vi "Add Element in Array Guidance.vi"(8 "error in (no error)":errorcluster, 10 "Guidance input":refnum<class "Guidance.lvclass">, 11 "Vessel in":refnum<class "Vessel.lvclass">) -> (0 "error out":errorcluster, 2 "Index":i32, 3 "Vessel out":refnum<class "Vessel.lvclass">)   [LabVIEW 2014, in "Vessel.lvclass"]
uses:
  Vessel.lvclass
  Guidance/Guidance.lvclass
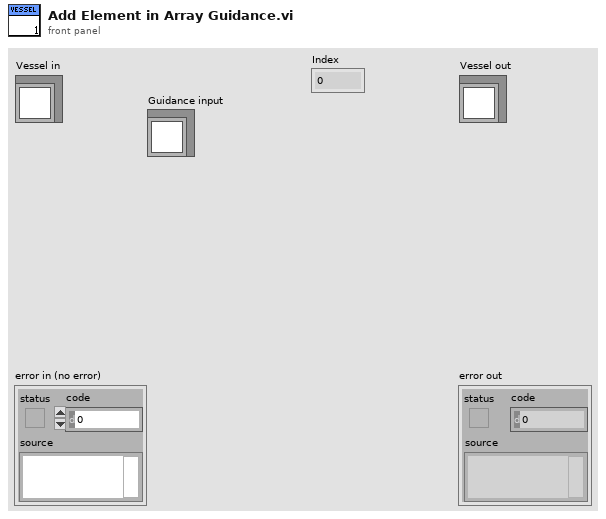
[diagram p1: front panel]
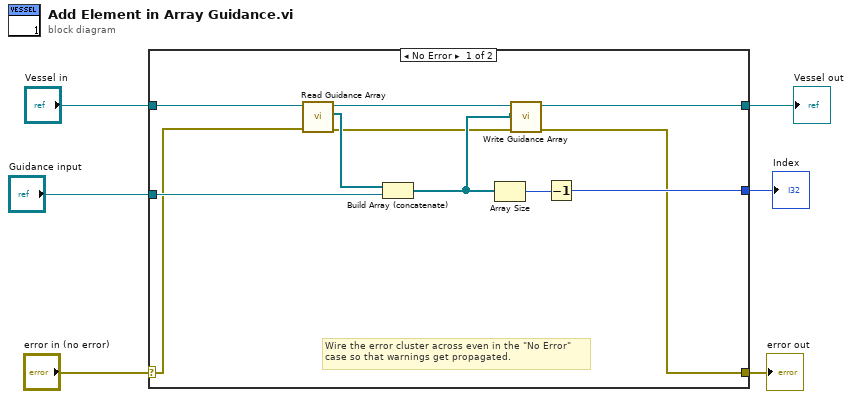
[diagram p0: block diagram]
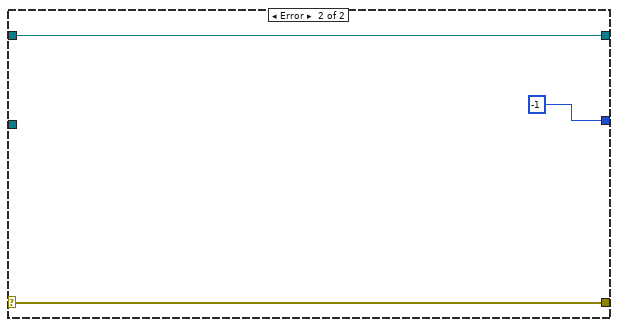
[diagram p2: hidden frame]
diagram:
  n1 = case shown="No Error" "error in (no error)" {
    selector: "error in (no error)" -> [w13 w20]
    tunnel: [w8 w20] -> w5
    tunnel: [w9 w19] -> w3
    tunnel: "Vessel in" -> [w14 w19]
    tunnel: "Guidance input" -> [w17 _]
    tunnel: [w15 -1] -> w2
    frame No Error {
      # "Wire the error cluster across even in the \"No Error\"\ncase so that warnings get propagated."
      n2 = call "Read Guidance Array.vi"("error in (no error)"=w13, "Vessel in"=w14) -> ("error out"=w7:errorcluster, "Guidance Array"=w11:refnum<class "Guidance.lvclass">[], "Vessel out"=w12:refnum<class "Vessel.lvclass">)  [unwired: 7 in]
      n3 = Build Array (concatenate)(w11, w17) -> (w10:refnum<class "Guidance.lvclass">[])
      n4 = Array Size(array=w10) -> (size(s)=w16:i32)
      n5 = call "Write Guidance Array.vi"("error in (no error)"=w7, "Guidance Array"=w10, "Vessel in"=w12) -> ("error out"=w8:errorcluster, "Vessel out"=w9:refnum<class "Vessel.lvclass">)  [unwired: 7 in]
      n6 = Decrement(x=w16) -> (x-1=w15:i32)
    }
    frame Error {
    }
  }
  "error out" <- w5
  "Vessel out" <- w3
  "Index" <- w2
